vi "Actor Core.vi"(8 "error in":errorcluster, 11 "DataBase in":refnum<class "DataBase.lvclass">) -> (0 "error out":errorcluster, 3 "Actor out":refnum<class "Actor.lvclass">)   [LabVIEW 2019, in "DataBase.lvlib" / "DataBase.lvclass"]
doc: "(<B>Filename</B>: Actor Framework.lvlib:Actor.lvclass:Actor Core.vi)\n\nReceives messages to the actor, reacts to them, and initiates any error handling that may shut the actor down.\n\nDescendant classes may override this VI to append parallel tasks for the actor to complete while it handles messages. Overrides use the Call Parent Class Method node."
uses:
  DataBase.lvclass
  C:/Program Files (x86)/National Instruments/LabVIEW 2019/vi.lib/ActorFramework/Actor/Actor.lvclass
  <vilib>/ActorFramework/Actor/Actor.lvclass
  DataBase.lvclass/DataBase.ctl
  <vilib>/ActorFramework/Actor/Actor.lvclass/Actor.ctl
  <vilib>/ActorFramework/Message Enqueuer/Message Enqueuer.lvclass/Message Enqueuer.ctl
  <vilib>/ActorFramework/Message Enqueuer/Init from Existing Queue.vi
  <vilib>/ActorFramework/Message Enqueuer/Enqueue.vi
  DataBase Messages/SelectData Msg/SelectData Msg.lvclass
  C:/Program Files (x86)/National Instruments/LabVIEW 2019/vi.lib/ActorFramework/Message/Message.lvclass
  DataBase Messages/NextPage Msg/NextPage Msg.lvclass
  DataBase Messages/PreviousPage Msg/PreviousPage Msg.lvclass
  DataBase Messages/Export Msg/Export Msg.lvclass
  DataBase Messages/SearchSerialNumber Msg/SearchSerialNumber Msg.lvclass
  DataBase Messages/ShowDetailResult Msg/ShowDetailResult Msg.lvclass
  <vilib>/ActorFramework/Message Priority Queue/Priority Enqueue.vi
  <vilib>/NI/Event Source Actor/Event Source/Event Source/Event Source.lvclass
  <vilib>/ActorFramework/Message Enqueuer/Message Enqueuer.lvclass
panel:
  in  "Station":T1(ring)
  in  "TableName":string(combo)
  in  "Radio Buttons":enum32{"PDF", "Excel"}(radio)=enum."Excel"
  in  "ShowDetail":bool
  in  "Search":bool
  in  "SerialNumber":string
  in  "TimeRange":T2(ring)
  in  "Export":bool
  in  "StartTime":timestamp=timestamp(3714617125.102728 s since 1904-01-01) format="%<%x>T"
  in  "PreviousPage":bool
  in  "NextPage":bool
  in  "Multicolumn Listbox":i32(listbox)
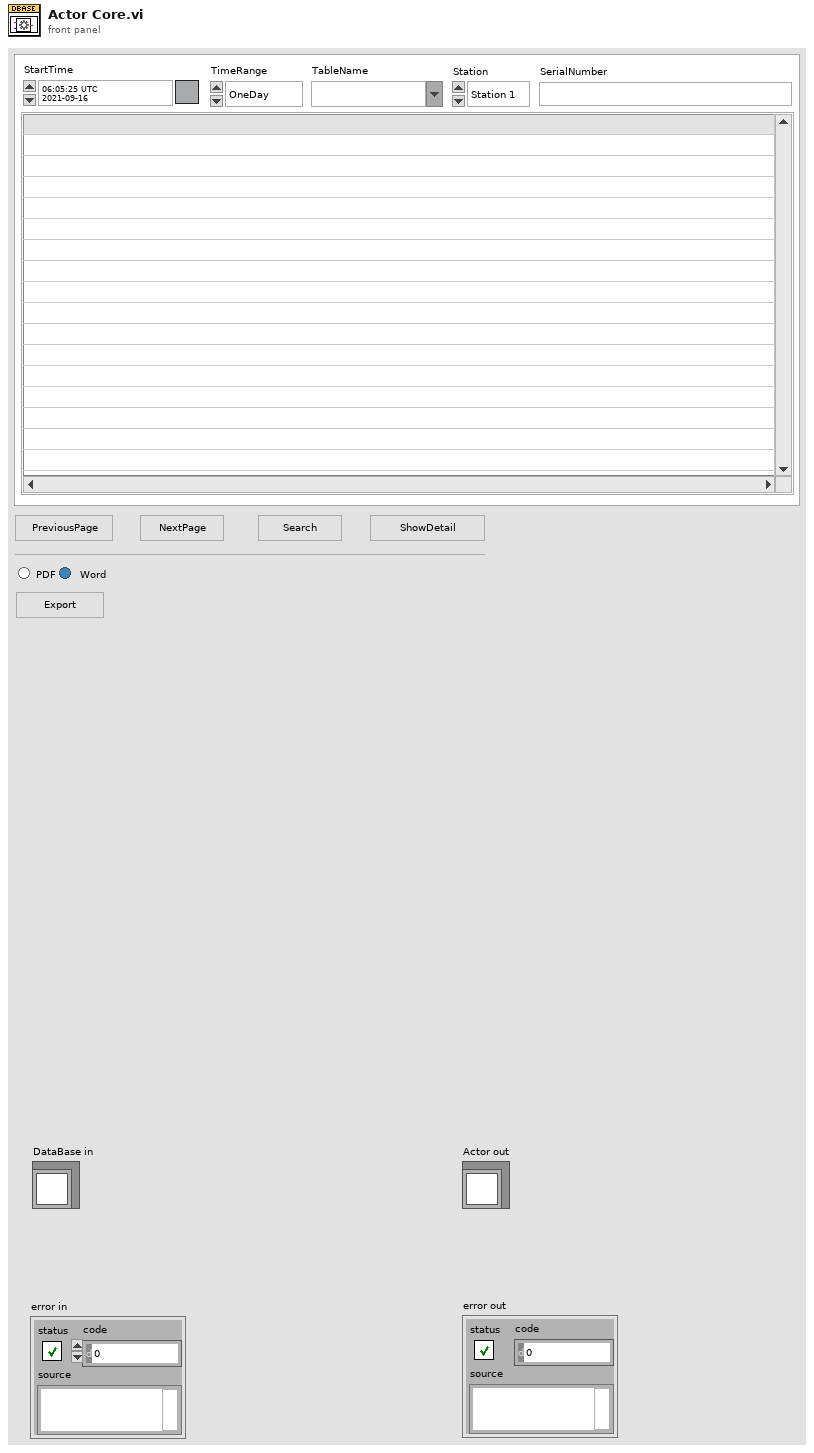
[diagram p1: front panel]
types:
  T1 = enum16{"Station 1", "Station 2", "Station 3", "Station 4"}
  T2 = enum16{"OneDay", "OneWeek", "OneMonth", "OneYear"}
  T3 = enum32{"Invalid", "Standard", "Closed", "Hidden", "Minimized", "Maximized"}
  T4 = enum32{"invalid app kind", "Development System", "Run Time System", "Student Edition", "Embedded LabVIEW", "Evaluation", "Custom"}
  T5 = cluster{"Core":cluster{"Current VI Reference":refnum<vi>, "Close Panel on Exit?":bool}, "Your Boolean data":bool, "Your string data":string}
  T6 = cluster{"Current VI Reference":refnum<vi>, "Close Panel on Exit?":bool}
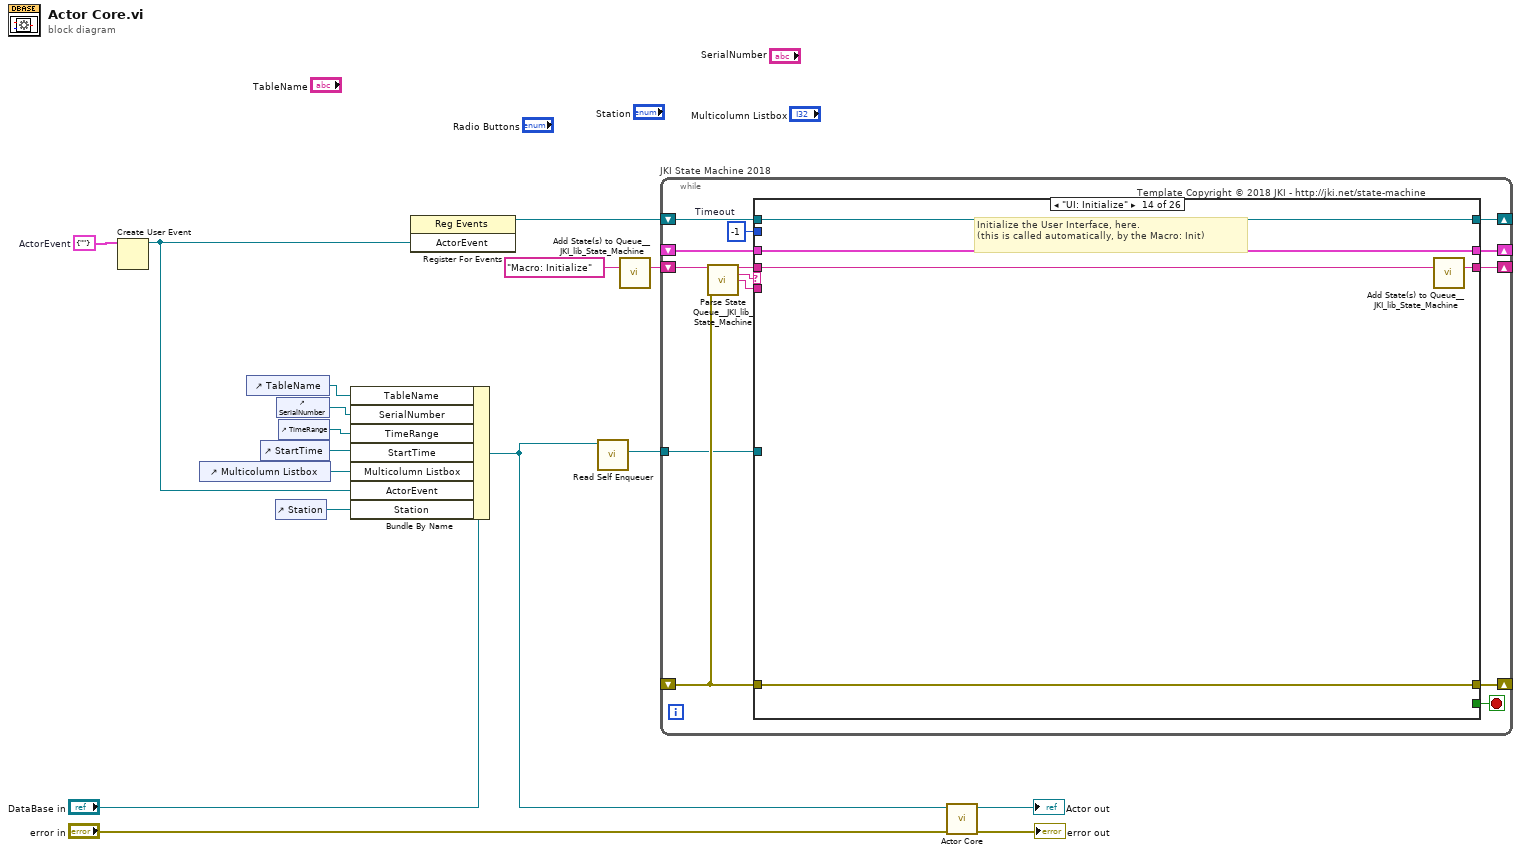
[diagram p0: block diagram]
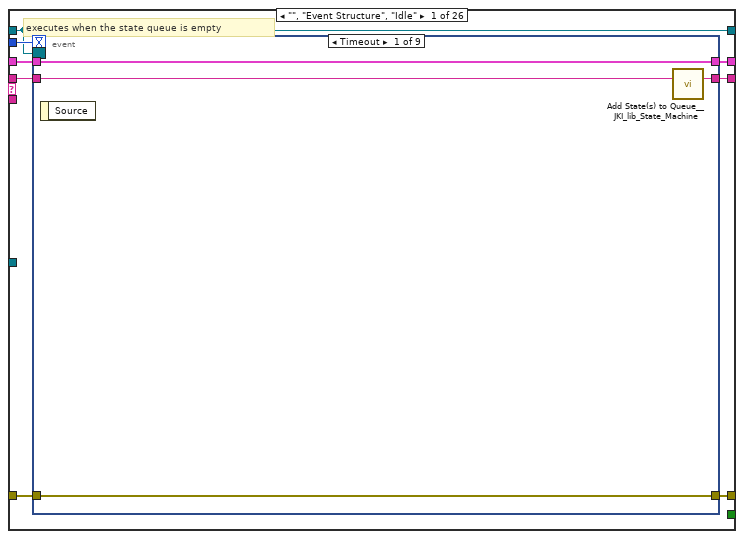
[diagram p2: hidden frame]
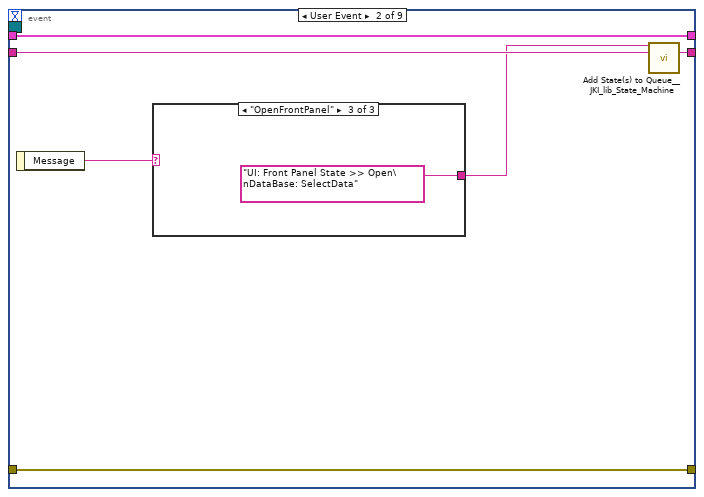
[diagram p3: hidden frame]
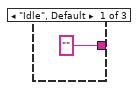
[diagram p4: hidden frame]
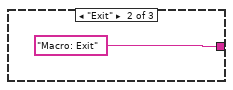
[diagram p5: hidden frame]
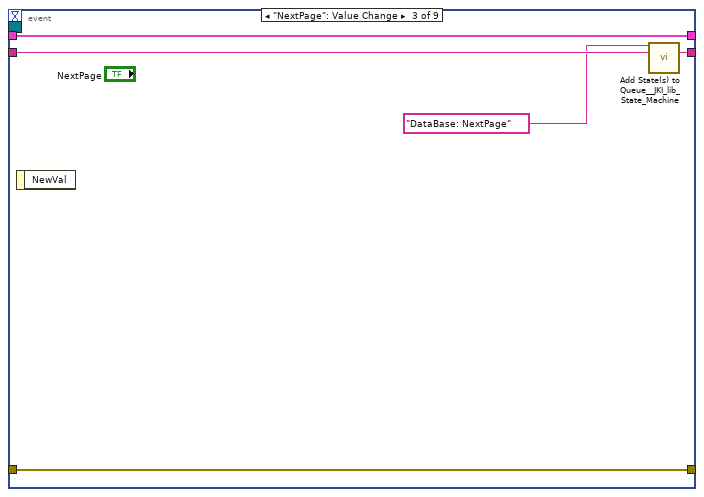
[diagram p6: hidden frame]
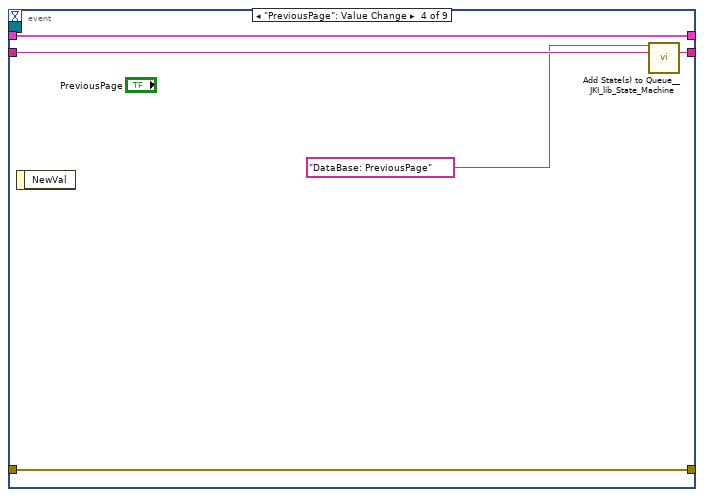
[diagram p7: hidden frame]
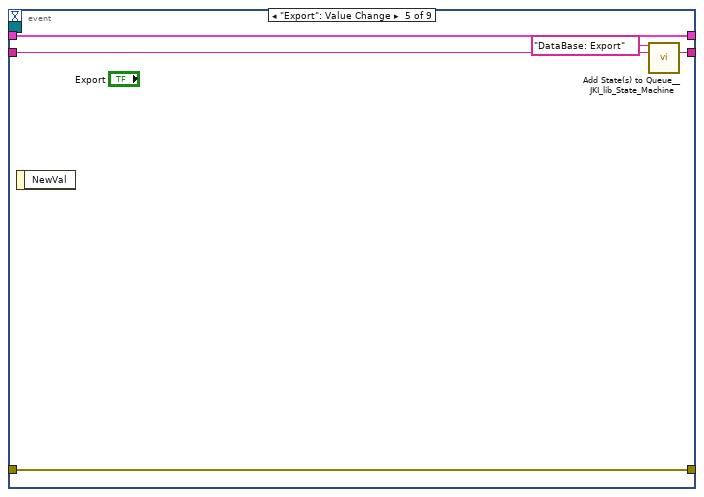
[diagram p8: hidden frame]
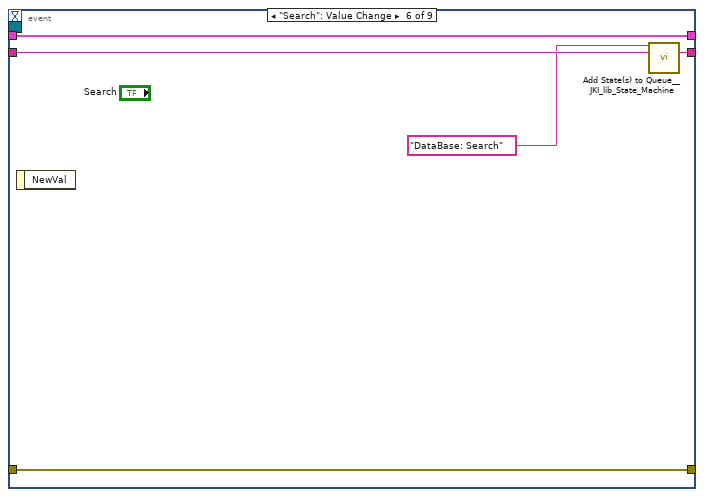
[diagram p9: hidden frame]
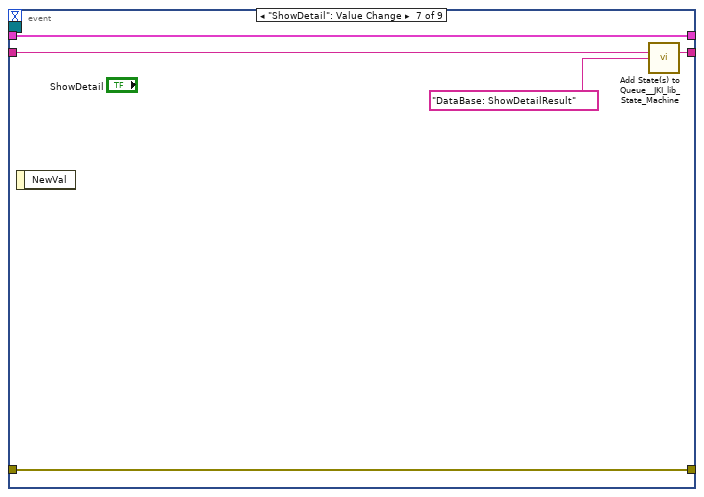
[diagram p10: hidden frame]
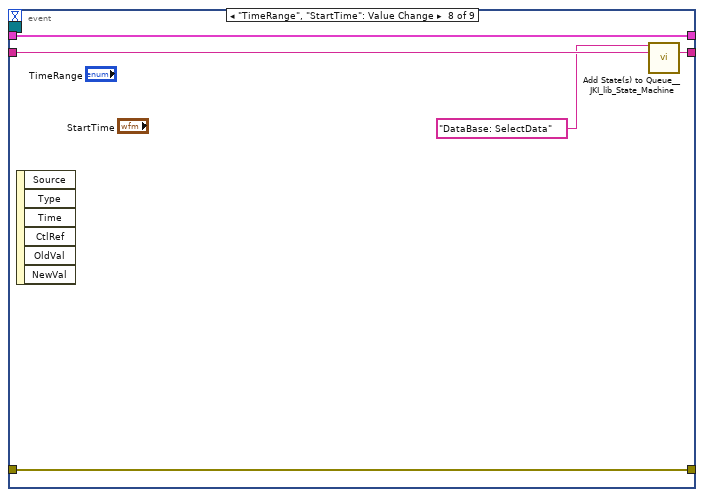
[diagram p11: hidden frame]
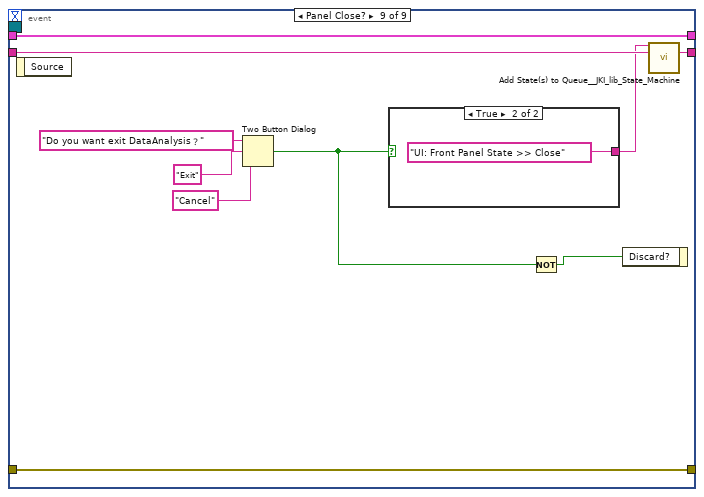
[diagram p12: hidden frame]
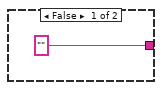
[diagram p13: hidden frame]
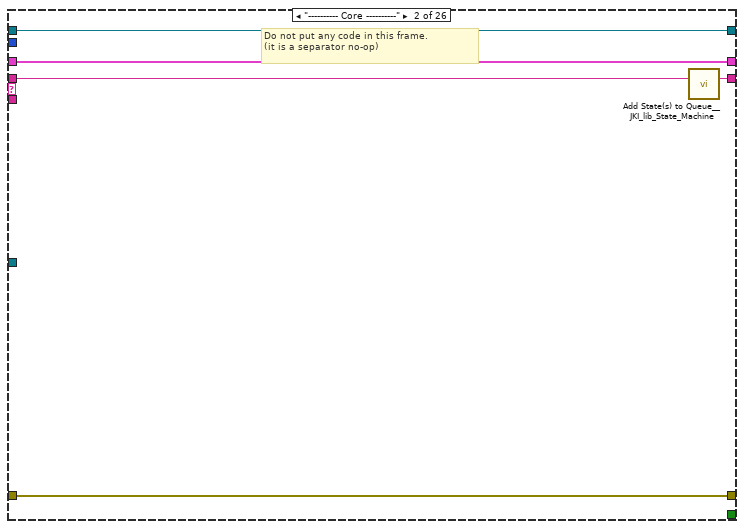
[diagram p14: hidden frame]
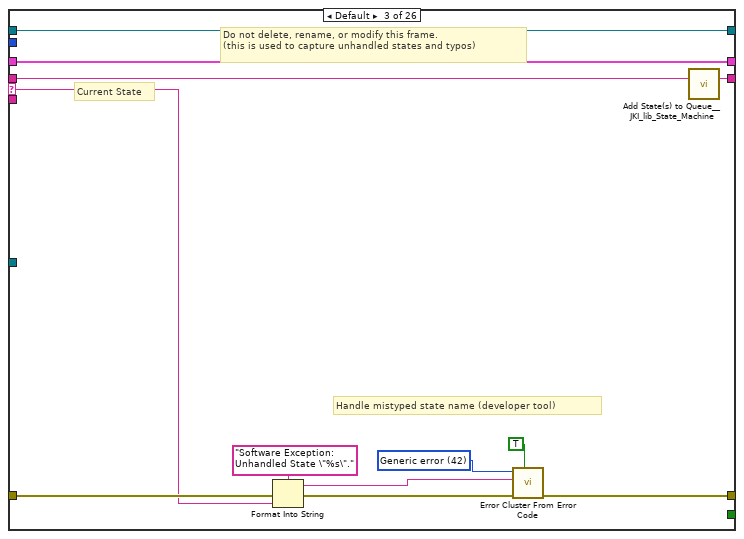
[diagram p15: hidden frame]
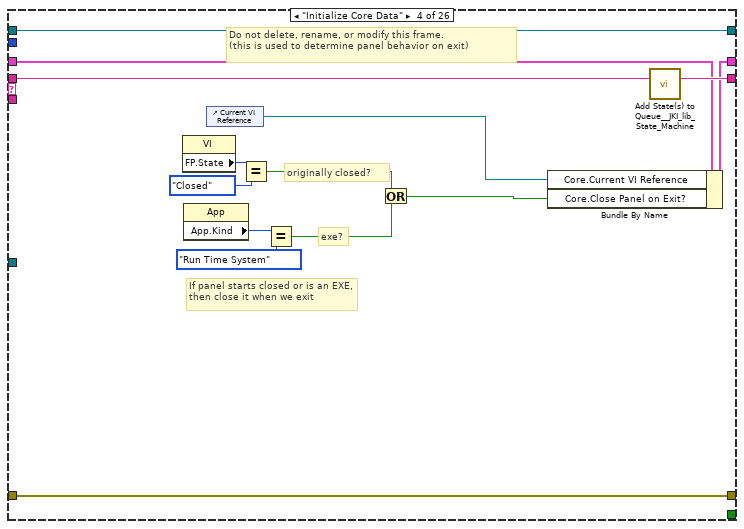
[diagram p16: hidden frame]
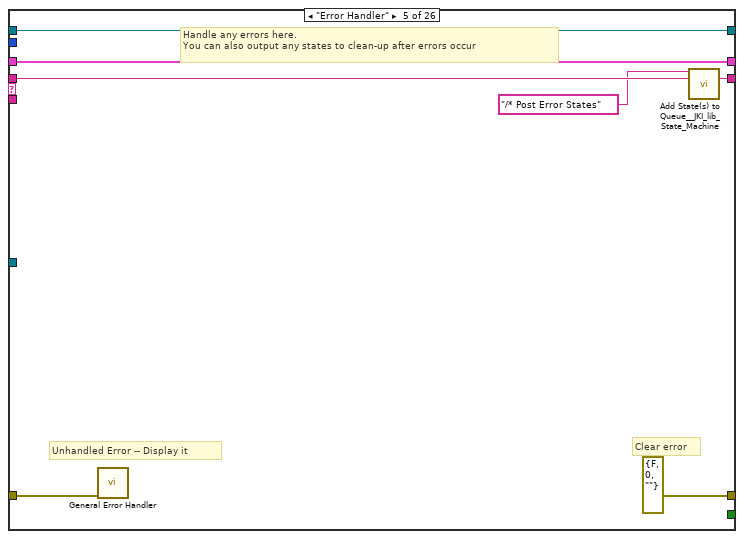
[diagram p17: hidden frame]
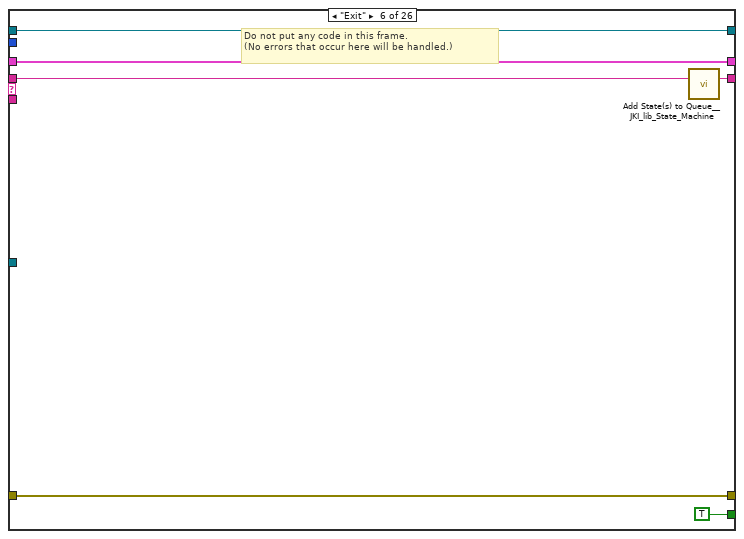
[diagram p18: hidden frame]
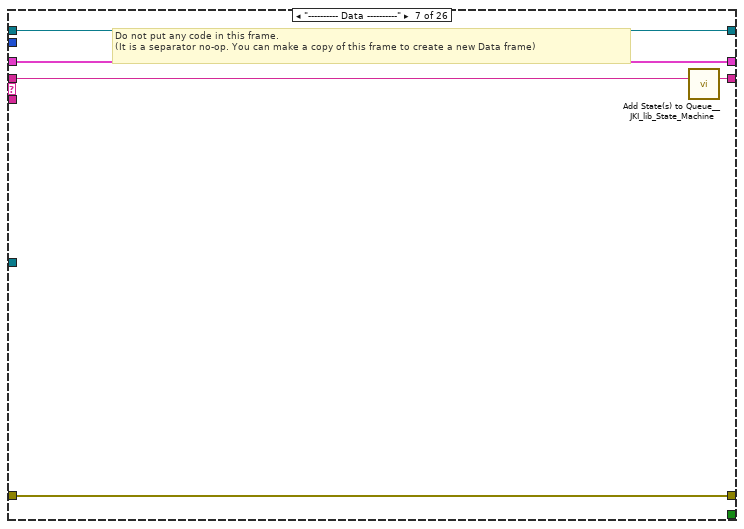
[diagram p19: hidden frame]
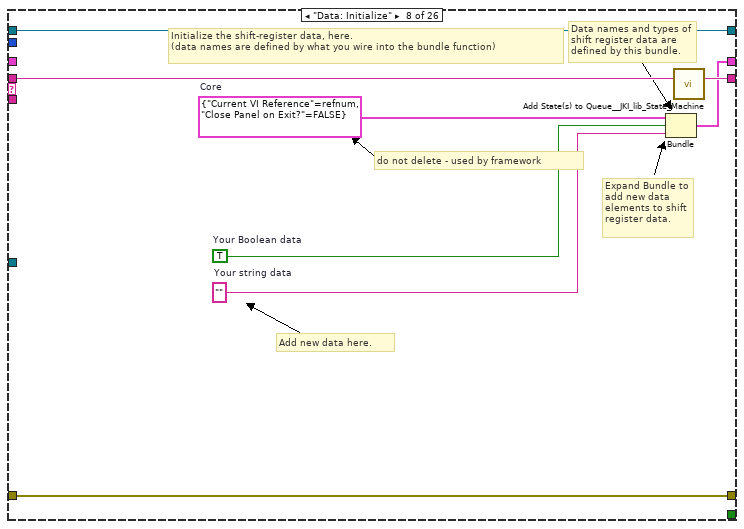
[diagram p20: hidden frame]
diagram:
  w11 = cluster{"Message":string} {"Message"=""}  # ActorEvent
  n1 = Create User Event(user event datatype=w11) -> (user event=w9:refnum<user-event>)  [unwired: 1 in, 1 out]
  n2 = control-ref of="Multicolumn Listbox"() -> (w7:refnum<vi>)
  n3 = control-ref of="TableName"() -> (w2:refnum<vi>)
  n4 = control-ref of="StartTime"() -> (w6:refnum<vi>)
  n5 = control-ref of="Station"() -> (w1:refnum<vi>)
  n6 = control-ref of="SerialNumber"() -> (w3:refnum<vi>)
  n7 = control-ref of="TimeRange"() -> (w5:refnum<vi>)
  n8 = Bundle By Name(cluster="DataBase in", "TableName"=w2, "SerialNumber"=w3, "TimeRange"=w5, "StartTime"=w6, "Multicolumn Listbox"=w7, "ActorEvent"=w9, "Station"=w1) -> (w4:refnum<class "DataBase.lvclass">)
  n9 = register-events(w9) -> (reference out=w12:refnum<event-registration>)  [unwired: 2 in, 1 out]
  n10 = call <vilib>:"Read Self Enqueuer.vi"("Actor"=w4) -> ("Self Enqueuer"=w8:refnum<class "Message Enqueuer.lvclass">)  [unwired: 10 in]
  n11 = call <vilib>:"Add State(s) to Queue__JKI_lib_State_Machine.vi"("State(s) in (\"\")"="Macro: Initialize") -> ("States Out"=w14:string)  [unwired: 14 in]
  n12 = while "JKI State Machine 2018" {
    shift-right: [w24] -> _
    shift-left: _ -> [w23]
    shift-right: [w27] -> _
    shift-left: _ -> [w21]
    shift-right: [w26] -> _
    shift-left: w14 -> [w28]
    shift-right: [w20] -> _
    shift-left: w12 -> [w19]
    tunnel: w8 -> [w18]
    stop <- w25 stop-if-true
    w22 = -1  # Timeout
    # "Template Copyright © 2018 JKI - http://jki.net/state-machine"
    n13 = call <vilib>:"Parse State Queue__JKI_lib_State_Machine.vi"("State Queue"=w28, "Error In (no error)"=w21) -> ("Remaining States"=w30:string, "Current State"=w31:string, "Arguments"=w29:string)  [unwired: 11 in]
    n14 = case shown="\"UI: Initialize\"" w31 {
      selector: w31 -> [_ _ w101 _ _ _ _ _ _ _ _ _ _ _ _ _ _ _ _ _ _ _ _ _ _ _]
      tunnel: w30 -> [w39 w99 w105 w125 w132 w138 w143 w151 w158 w163 w168 w174 w179 w184 w191 w203 w273 w279 w290 w295 w302 w308 w314 w320 w326 w332]
      tunnel: w29 -> [_ _ _ _ _ _ _ _ _ _ _ _ _ _ w186 w197 _ _ _ _ _ _ _ _ _ _]
      tunnel: w23 -> [w37 w96 w103 w118 w129 w136 w140 _ w153 w160 w166 w172 w176 w182 w189 w199 w270 w276 w287 w292 w300 w305 w311 w317 w323 w329]
      tunnel: [w36 w97 w107 w122 errorcluster {"status"=FALSE, "code"=0, "source"=""} ("error out") w135 w141 w148 w154 w161 w165 w169 w177 w181 w187 w200 w271 w277 w288 w293 w297 w306 w312 w318 w324 w330] -> w27
      tunnel: w21 -> [w35 w97 w106 w122 w128 w135 w141 w148 w155 w161 w165 w170 w177 w181 w188 w201 w271 w277 w288 w293 w297 w306 w312 w318 w324 w330]
      tunnel: [w38 w98 w104 w124 w131 w137 w142 w150 w157 w162 w167 w173 w178 w183 w190 w202 w272 w278 w289 w294 w301 w307 w313 w319 w325 w331] -> w26
      tunnel: [_ _ _ _ _ TRUE _ _ _ _ _ _ _ _ _ _ _ _ _ _ _ _ _ _ _ _] -> w25
      tunnel: [w34 w96 w103 w123 w129 w136 w140 w149 w153 w160 w166 w172 w176 w182 w189 w199 w270 w276 w287 w292 w300 w305 w311 w317 w323 w329] -> w24
      tunnel: w22 -> [w33 _ _ _ _ _ _ _ _ _ _ _ _ _ _ _ _ _ _ _ _ _ _ _ _ _]
      tunnel: [w32 w95 w100 w112 w126 w133 w139 w144 w152 w159 w164 w171 w175 w180 w185 w196 w269 w274 w280 w291 w299 w304 w310 w316 w322 w328] -> w20
      tunnel: w19 -> [w32 w95 w100 w112 w126 w133 w139 w144 w152 w159 w164 w171 w175 w180 w185 w196 w269 w274 w280 w291 w299 w304 w310 w316 w322 w328]
      tunnel: w18 -> [_ _ _ _ _ _ _ _ _ _ _ _ _ _ _ _ _ _ _ _ w298 w303 w309 w315 w321 w327]
      frame "", "Event Structure", "Idle" {
        # "executes when the state queue is empty"
        n15 = event shown="[0] Timeout" {
          selector: w32 -> [_ _ _ _ _ _ _ _ _]
          dyn-events: _ -> [_ _ _ _ _ _ _ _ _]
          timeout: w33 -> [_ _ _ _ _ _ _ _ _]
          tunnel: w39 -> [w43 w49 w57 w62 w67 w72 w77 w82 w92]
          tunnel: [w42 w48 w56 w61 w66 w71 w76 w81 w91] -> w38
          tunnel: w37 -> [w40 w46 w54 w59 w64 w69 w74 w79 w89]
          tunnel: [w41 w47 w55 w60 w65 w70 w75 w80 w90] -> w36
          tunnel: w35 -> [w41 w47 w55 w60 w65 w70 w75 w80 w90]
          tunnel: [w40 w46 w54 w59 w64 w69 w74 w79 w89] -> w34
          event Timeout {
            n16 = event-data() -> ()  [unwired: 1 in, 1 out]
            n17 = call <vilib>:"Add State(s) to Queue__JKI_lib_State_Machine.vi"("State(s) in (\"\")"=w43) -> ("States Out"=w42:string)  [unwired: 14 in]
          }
          event User Event {
            n18 = event-data() -> ("Message"=w45:string)  [unwired: 1 in]
            n19 = case shown="\"OpenFrontPanel\"" w45 {
              tunnel: ["" "Macro: Exit" "UI: Front Panel State >> Open\nDataBase: SelectData"] -> w44
              frame "Idle", Default {
              }
              frame "Exit" {
              }
              frame "OpenFrontPanel" {
              }
            }
            n20 = call <vilib>:"Add State(s) to Queue__JKI_lib_State_Machine.vi"("State(s) in Front (\"\")"=w44, "State(s) in (\"\")"=w49) -> ("States Out"=w48:string)  [unwired: 13 in]
          }
          event "NextPage": Value Change {
            n21 = event-data() -> ()  [unwired: 1 in, 1 out]
            n22 = call <vilib>:"Add State(s) to Queue__JKI_lib_State_Machine.vi"("State(s) in Front (\"\")"="DataBase: NextPage" ("State(s) in Front (\"\")"), "State(s) in (\"\")"=w57) -> ("States Out"=w56:string)  [unwired: 13 in]
          }
          event "PreviousPage": Value Change {
            n23 = event-data() -> ()  [unwired: 1 in, 1 out]
            n24 = call <vilib>:"Add State(s) to Queue__JKI_lib_State_Machine.vi"("State(s) in Front (\"\")"="DataBase: PreviousPage" ("State(s) in Front (\"\")"), "State(s) in (\"\")"=w62) -> ("States Out"=w61:string)  [unwired: 13 in]
          }
          event "Export": Value Change {
            n25 = event-data() -> ()  [unwired: 1 in, 1 out]
            n26 = call <vilib>:"Add State(s) to Queue__JKI_lib_State_Machine.vi"("State(s) in Front (\"\")"="DataBase: Export" ("State(s) in Front (\"\")"), "State(s) in (\"\")"=w67) -> ("States Out"=w66:string)  [unwired: 13 in]
          }
          event "Search": Value Change {
            n27 = event-data() -> ()  [unwired: 1 in, 1 out]
            n28 = call <vilib>:"Add State(s) to Queue__JKI_lib_State_Machine.vi"("State(s) in Front (\"\")"="DataBase: Search" ("State(s) in Front (\"\")"), "State(s) in (\"\")"=w72) -> ("States Out"=w71:string)  [unwired: 13 in]
          }
          event "ShowDetail": Value Change {
            n29 = event-data() -> ()  [unwired: 1 in, 1 out]
            n30 = call <vilib>:"Add State(s) to Queue__JKI_lib_State_Machine.vi"("State(s) in (\"\")"=w77, "State(s) at Back (\"\")"="DataBase: ShowDetailResult" ("State(s) at Back (\"\")")) -> ("States Out"=w76:string)  [unwired: 13 in]
          }
          event "TimeRange", "StartTime": Value Change {
            n31 = event-data() -> ()  [unwired: 1 in, 6 out]
            n32 = call <vilib>:"Add State(s) to Queue__JKI_lib_State_Machine.vi"("State(s) in Front (\"\")"="DataBase: SelectData" ("State(s) in Front (\"\")"), "State(s) in (\"\")"=w82) -> ("States Out"=w81:string)  [unwired: 13 in]
          }
          event Panel Close? {
            n33 = event-data() -> ()  [unwired: 1 in, 1 out]
            n34 = Two Button Dialog(message="Do you want exit DataAnalysis？", 1:"Cancel" ("F button name (\"Cancel\")"), 2:"Exit" ("T button name (\"OK\")")) -> (T button?=w86:bool)
            n35 = case shown="True" w86 {
              tunnel: ["" "UI: Front Panel State >> Close"] -> w83
              frame False {
              }
              frame True {
              }
            }
            n36 = Not(x=w86) -> (.not. x?=w84:bool)
            n37 = event-data("Discard?"=w84) -> ()  [unwired: 1 in, 1 out]
            n38 = call <vilib>:"Add State(s) to Queue__JKI_lib_State_Machine.vi"("State(s) in Front (\"\")"=w83, "State(s) in (\"\")"=w92) -> ("States Out"=w91:string)  [unwired: 13 in]
          }
        }
      }
      frame "---------- Core ----------" {
        # "Do not put any code in this frame.\n(it is a separator no-op)"
        n39 = call <vilib>:"Add State(s) to Queue__JKI_lib_State_Machine.vi"("State(s) in (\"\")"=w99) -> ("States Out"=w98:string)  [unwired: 14 in]
      }
      frame Default {
        w110 = 42 items=["No error", "Argument error", "Memory is full", "Out of zone", "End of file", "File already open", "Generic file I/O error", "File not found", "File permission error", "Disk is full", "Duplicate path", "Too many files open", "System feature not enabled", "Resource file not found", "Cannot add resource", "Resource not found", "Image not found", "Image memory error", "Pen does not exist", "Config type invalid", "Config token not found", "Config parse error", "Config memory error", "Bad external code format", "Bad external code offset", "External code not present", "Null window", "Destroy window error", "Null menu", "Print aborted", "Bad print record", "Print driver error", "Windows error during printing", "Memory error during printing", "Print dialog error", "Generic print error", "Invalid device refnum", "Device not found", "Device parameter error", "Device unit error", "Cannot open device", "Device call aborted", "Generic error", "Cancelled by user", "Object ID too low", "Object ID too high", "Object not in heap", "Unknown heap", "Unknown object (invalid DefProc)", "Unknown object (DefProc not in table)", "Message out of range", "Invalid (null) method", "Unknown message", "Manager call not supported", "Bad address", "Network operation in progress", "Network operation timed out", "Connection is busy", "Network attribute not supported", "Network error", "Address in use", "System out of memory", "Connection aborted", "Connection refused", "Not connected", "Already connected", "Connection closed", "Initialization error (interapplication manager)", "Bad occurrence", "Wait on unbound occurrence handler", "Occurrence queue overflow", "Datalog type conflict", "Unused", "Unrecognized type (interapplication manager)", "Memory corrupt", "Failed to make temporary DLL", "Old CIN version", "Drag socket not found", "Failed to load drop-object", "Failed to register OLE object", "Failed to release OLE object", "Format specifier type mismatch", "Unknown format specifier", "Too few format specifiers", "Too many format specifiers", "Scan failed", "Newer CIN version", "Error converting to variant", "Runtime menu error", "Password tampered", "Variant attribute not found", "Incompatible variant data type", "Event data is not available", "Event Store is not present", "Occurrence is not found", "Event Queue is not created", "Event info is not available", "Refnum passed is NULL", "Error retrieving Class GUID", "Error retrieving CoClass GUID", "Error retrieving TypeLib GUID.", "Bad built application magic bytes.", "Specific driver is different from the specific driver associated with the Logical Name.", "There is no session opened to the class driver.", "Max Error", "MAX - Error with config objects", "MAX - Error loading configuration", "MAX - Group not supported"]
        # "Current State"
        # "Do not delete, rename, or modify this frame.\n(this is used to capture unhandled states and typos)"
        # "Handle mistyped state name (developer tool)"
        n40 = Format Into String(format string="Software Exception: Unhandled State \"%s\"." ("message"), error in=w106, w101) -> (resulting string=w109:string, error out=w108:errorcluster)  [unwired: 1 in]
        n41 = call <vilib>:"Error Cluster From Error Code.vi"("show call chain? (False)"=TRUE, "error in (no error)"=w108, "error message (\"\")"=w109, "error code (0)"=w110) -> ("error out"=w107:errorcluster)  [unwired: 5 in]
        n42 = call <vilib>:"Add State(s) to Queue__JKI_lib_State_Machine.vi"("State(s) in (\"\")"=w105) -> ("States Out"=w104:string)  [unwired: 14 in]
      }
      frame "Initialize Core Data" {
        # "Do not delete, rename, or modify this frame.\n(this is used to determine panel behavior on exit)"
        # "originally closed?"
        # "exe?"
        # "If panel starts closed or is an EXE, then close it when we exit"
        n43 = property class="VI"() -> ("FP.State"=w115:T3)  [unwired: 2 in, 2 out]
        n44 = property class="App"() -> ("App.Kind"=w121:T4)  [unwired: 2 in, 2 out]
        n45 = control-ref of="Current VI Reference"() -> (w116:refnum<vi>)
        n46 = Equal?(x=w115, y=T3."Closed" ("Front Panel Window:State")) -> (x = y?=w113:bool)
        n47 = Equal?(x=w121, y=T4."Run Time System" ("Application:Kind")) -> (x = y?=w119:bool)
        n48 = Or(x=w113, y=w119) -> (x .or. y?=w117:bool)
        n49 = Bundle By Name(cluster=w118, "Core.Current VI Reference"=w116, "Core.Close Panel on Exit?"=w117) -> (w123:T5)
        n50 = call <vilib>:"Add State(s) to Queue__JKI_lib_State_Machine.vi"("State(s) in (\"\")"=w125) -> ("States Out"=w124:string)  [unwired: 14 in]
      }
      frame "Error Handler" {
        # "Unhandled Error -- Display it"
        # "Handle any errors here.\nYou can also output any states to clean-up after errors occur"
        # "Clear error"
        n51 = call <vilib>:"General Error Handler.vi"("error in (no error)"=w128) -> ()  [unwired: 10 in, 5 out]
        n52 = call <vilib>:"Add State(s) to Queue__JKI_lib_State_Machine.vi"("State(s) in Front (\"\")"="/* Post Error States", "State(s) in (\"\")"=w132) -> ("States Out"=w131:string)  [unwired: 13 in]
      }
      frame "Exit" {
        # "Do not put any code in this frame.\n(No errors that occur here will be handled.)"
        n53 = call <vilib>:"Add State(s) to Queue__JKI_lib_State_Machine.vi"("State(s) in (\"\")"=w138) -> ("States Out"=w137:string)  [unwired: 14 in]
      }
      frame "---------- Data ----------" {
        # "Do not put any code in this frame.\n(It is a separator no-op. You can make a copy of this frame to create a new Data frame)"
        n54 = call <vilib>:"Add State(s) to Queue__JKI_lib_State_Machine.vi"("State(s) in (\"\")"=w143) -> ("States Out"=w142:string)  [unwired: 14 in]
      }
      frame "Data: Initialize" {
        w145 = T6 {"Current VI Reference"=refnum, "Close Panel on Exit?"=FALSE}  # Core
        w147 = TRUE  # Your Boolean data
        w146 = ""  # Your string data
        # "do not delete - used by framework"
        # "Expand Bundle to add new data elements to shift register data."
        # "Add new data here."
        # "Data names and types of shift register data are defined by this bundle."
        # "Initialize the shift-register data, here.\n(data names are defined by what you wire into the bundle function)"
        n55 = Bundle("Core"=w145, "Your Boolean data"=w147, "Your string data"=w146) -> (w149:T5)  [unwired: 1 in]
        n56 = call <vilib>:"Add State(s) to Queue__JKI_lib_State_Machine.vi"("State(s) in (\"\")"=w151) -> ("States Out"=w150:string)  [unwired: 14 in]
      }
      frame "Data: Cleanup" {
        # "Cleanup any data and references, here.\n(this is called automatically, by the Macro: Exit)"
        n57 = Unbundle By Name(w153) -> ("Core.Current VI Reference"=w156:refnum<vi>)
        n58 = Close Reference(reference=w156, error in (no error)=w155) -> (error out=w154:errorcluster)
        n59 = call <vilib>:"Add State(s) to Queue__JKI_lib_State_Machine.vi"("State(s) in (\"\")"=w158) -> ("States Out"=w157:string)  [unwired: 14 in]
      }
      frame "---------- Events ----------" {
        # "Do not put any code in this frame.\n(It is a separator no-op. You can make a copy of this frame to create a new UI frame)"
        n60 = call <vilib>:"Add State(s) to Queue__JKI_lib_State_Machine.vi"("State(s) in (\"\")"=w163) -> ("States Out"=w162:string)  [unwired: 14 in]
      }
      frame "Events: Register" {
        n61 = call <vilib>:"Add State(s) to Queue__JKI_lib_State_Machine.vi"("State(s) in (\"\")"=w168) -> ("States Out"=w167:string)  [unwired: 14 in]
      }
      frame "Events: Unregister" {
        # "Do not put any code in this frame.\n(It is a separator no-op. You can make a copy of this frame to create a new UI frame)"
        n62 = Unregister For Events(event registration refnum=w171, error in=w170) -> (error out=w169:errorcluster)
        n63 = call <vilib>:"Add State(s) to Queue__JKI_lib_State_Machine.vi"("State(s) in (\"\")"=w174) -> ("States Out"=w173:string)  [unwired: 14 in]
      }
      frame "---------- UI ----------" {
        # "Do not put any code in this frame.\n(It is a separator no-op. You can make a copy of this frame to create a new UI frame)"
        n64 = call <vilib>:"Add State(s) to Queue__JKI_lib_State_Machine.vi"("State(s) in (\"\")"=w179) -> ("States Out"=w178:string)  [unwired: 14 in]
      }
      frame "UI: Initialize" {
        # "Initialize the User Interface, here.\n(this is called automatically, by the Macro: Init)"
        n65 = call <vilib>:"Add State(s) to Queue__JKI_lib_State_Machine.vi"("State(s) in (\"\")"=w184) -> ("States Out"=w183:string)  [unwired: 14 in]
      }
      frame "UI: Cursor Set" {
        # "Argument"
        # "Set and Unset Cursor Busy.\n(Usage: \"UI: Cursor Set >> Busy|Idle\")"
        n66 = case shown="\"Idle\", Default" w186 {
          tunnel: w188 -> [w193 w195]
          tunnel: [w192 w194] -> w187
          frame "Idle", Default {
            n67 = call <vilib>:"Unset Busy.vi"("error in (no error)"=w193) -> ("error out"=w192:errorcluster)  [unwired: 10 in]
          }
          frame "Busy" {
            n68 = call <vilib>:"Set Busy.vi"("error in (no error)"=w195) -> ("error out"=w194:errorcluster)  [unwired: 9 in, 1 out]
          }
        }
        n69 = call <vilib>:"Add State(s) to Queue__JKI_lib_State_Machine.vi"("State(s) in (\"\")"=w191) -> ("States Out"=w190:string)  [unwired: 14 in]
      }
      frame "UI: Front Panel State" {
        # "Argument"
        # "Set Front Panel Open or Closed\n(Usage: \"UI: Front Panel State >> Open|Close\")"
        n70 = Unbundle By Name(w199) -> ("Core.Current VI Reference"=w198:refnum<vi>)
        n71 = case shown="\"Open\", \"Standard\", Default" w197 {
          tunnel: w201 -> [w209 w224 w235 w248 w261]
          tunnel: [w211 w225 w237 w250 w263] -> w200
          tunnel: w198 -> [w210 w222 w236 w249 w262]
          frame "Open", "Standard", Default {
            w204 = T3."Standard" ("State")
            n72 = property class="VI"(reference=w210, error in=w209) -> (reference out=w207:refnum<vi>, error out=w208:errorcluster, "FP.State"=w206:T3)
            n73 = Not Equal?(x=w206, y=w204) -> (x != y?=w205:bool)
            n74 = case shown="True" w205 {
              tunnel: [w215 w217] -> w211
              tunnel: w208 -> [w214 w217]
              tunnel: w207 -> [w213 _]
              tunnel: w204 -> [w212 _]
              frame True {
                n75 = invoke class="VI" method="FP.Open"(reference=w213, error in=w214, "Activate"=TRUE, "State"=w212) -> (error out=w215:errorcluster)  [unwired: 1 in, 4 out]
              }
              frame False {
              }
            }
          }
          frame "Close", "Closed" {
            n76 = property class="VI"(reference=w222, error in=w224) -> (reference out=w221:refnum<vi>, error out=w223:errorcluster, "FP.State"=w219:T3)
            n77 = Not Equal?(x=w219, y=T3."Closed" ("Front Panel Window:State")) -> (x != y?=w218:bool)
            n78 = case shown="True" w218 {
              tunnel: [w226 w229] -> w225
              tunnel: w223 -> [w226 w228]
              tunnel: w221 -> [_ w227]
              frame False {
              }
              frame True {
                n79 = invoke class="VI" method="FP.Close"(reference=w227, error in=w228) -> (error out=w229:errorcluster)  [unwired: 1 in, 2 out]
              }
            }
          }
          frame "Hidden", "Hide" {
            w230 = T3."Hidden" ("State")
            n80 = property class="VI"(reference=w236, error in=w235) -> (reference out=w233:refnum<vi>, error out=w234:errorcluster, "FP.State"=w232:T3)
            n81 = Not Equal?(x=w232, y=w230) -> (x != y?=w231:bool)
            n82 = case shown="True" w231 {
              tunnel: [w241 w242] -> w237
              tunnel: w234 -> [w240 w242]
              tunnel: w233 -> [w239 _]
              tunnel: w230 -> [w238 _]
              frame True {
                n83 = invoke class="VI" method="FP.Open"(reference=w239, error in=w240, "State"=w238) -> (error out=w241:errorcluster)  [unwired: 2 in, 4 out]
              }
              frame False {
              }
            }
          }
          frame "Minimize", "Minimized" {
            w243 = T3."Minimized" ("State")
            n84 = property class="VI"(reference=w249, error in=w248) -> (reference out=w246:refnum<vi>, error out=w247:errorcluster, "FP.State"=w245:T3)
            n85 = Not Equal?(x=w245, y=w243) -> (x != y?=w244:bool)
            n86 = case shown="True" w244 {
              tunnel: [w254 w255] -> w250
              tunnel: w247 -> [w253 w255]
              tunnel: w246 -> [w252 _]
              tunnel: w243 -> [w251 _]
              frame True {
                n87 = invoke class="VI" method="FP.Open"(reference=w252, error in=w253, "State"=w251) -> (error out=w254:errorcluster)  [unwired: 2 in, 4 out]
              }
              frame False {
              }
            }
          }
          frame "Maximize", "Maximized" {
            w256 = T3."Maximized" ("State")
            n88 = property class="VI"(reference=w262, error in=w261) -> (reference out=w259:refnum<vi>, error out=w260:errorcluster, "FP.State"=w258:T3)
            n89 = Not Equal?(x=w258, y=w256) -> (x != y?=w257:bool)
            n90 = case shown="True" w257 {
              tunnel: [w267 w268] -> w263
              tunnel: w260 -> [w266 w268]
              tunnel: w259 -> [w265 _]
              tunnel: w256 -> [w264 _]
              frame True {
                n91 = invoke class="VI" method="FP.Open"(reference=w265, error in=w266, "State"=w264) -> (error out=w267:errorcluster)  [unwired: 2 in, 4 out]
              }
              frame False {
              }
            }
          }
        }
        n92 = call <vilib>:"Add State(s) to Queue__JKI_lib_State_Machine.vi"("State(s) in (\"\")"=w203) -> ("States Out"=w202:string)  [unwired: 14 in]
      }
      frame "---------- Macro ----------" {
        # "Do not put any code in this frame.\n(It is a separator no-op. You can make a copy of this frame to create a new Macro frame)"
        n93 = call <vilib>:"Add State(s) to Queue__JKI_lib_State_Machine.vi"("State(s) in (\"\")"=w273) -> ("States Out"=w272:string)  [unwired: 14 in]
      }
      frame "Macro: Initialize" {
        # "Initialization Macro\n(This is called once, when the VI starts)"
        n94 = call <vilib>:"Add State(s) to Queue__JKI_lib_State_Machine.vi"("State(s) in Front (\"\")"="Data: Initialize\nInitialize Core Data\nEvents: Register\nUI: Initialize\nUI: Front Panel State >> Closed", "State(s) in (\"\")"=w279) -> ("States Out"=w278:string)  [unwired: 13 in]
      }
      frame "Macro: Exit" {
        # "Exit Macro\n(This is called once, when the VI exits)"
        n95 = Unbundle By Name(w287) -> ("Core.Close Panel on Exit?"=w286:bool)
        n96 = Select(t="UI: Front Panel State >> Close", s=w286, f="") -> (s? t:f=w283:string)
        n97 = call <vilib>:"Add State(s) to Queue__JKI_lib_State_Machine.vi"("State(s) in (\"\")"=w283, "State(s) at Back (\"\")"="Data: Cleanup\nEvents: Unregister\nExit") -> ("States Out"=w281:string)  [unwired: 13 in]
        n98 = call <vilib>:"Add State(s) to Queue__JKI_lib_State_Machine.vi"("State(s) in Front (\"\")"=w281, "State(s) in (\"\")"=w290) -> ("States Out"=w289:string)  [unwired: 13 in]
      }
      frame "---------- DataBase ----------" {
        # "Template Separator\n(You can make a copy of, or modify, this frame)"
        n99 = call <vilib>:"Add State(s) to Queue__JKI_lib_State_Machine.vi"("State(s) in (\"\")"=w295) -> ("States Out"=w294:string)  [unwired: 14 in]
      }
      frame "DataBase: SelectData" {
        # "Your code here.\n(You can make a copy of, or modify, this frame)"
        n100 = property on="Multicolumn Listbox" class="MCListbox (strict)"(error in=w297, "Value"=-1 ("Multicolumn Listbox")) -> ()  [unwired: 1 in, 2 out]
        n101 = call "Send SelectData.vi"("Message Enqueuer"=w298) -> ()  [unwired: 9 in, 2 out]
        n102 = call <vilib>:"Add State(s) to Queue__JKI_lib_State_Machine.vi"("State(s) in (\"\")"=w302) -> ("States Out"=w301:string)  [unwired: 14 in]
      }
      frame "DataBase: NextPage" {
        n103 = call "Send NextPage.vi"("Message Enqueuer"=w303) -> ()  [unwired: 9 in, 2 out]
        n104 = call <vilib>:"Add State(s) to Queue__JKI_lib_State_Machine.vi"("State(s) in (\"\")"=w308) -> ("States Out"=w307:string)  [unwired: 14 in]
      }
      frame "DataBase: PreviousPage" {
        n105 = call "Send PreviousPage.vi"("Message Enqueuer"=w309) -> ()  [unwired: 9 in, 2 out]
        n106 = call <vilib>:"Add State(s) to Queue__JKI_lib_State_Machine.vi"("State(s) in (\"\")"=w314) -> ("States Out"=w313:string)  [unwired: 14 in]
      }
      frame "DataBase: Export" {
        n107 = call "Send Export.vi"("Message Enqueuer"=w315) -> ()  [unwired: 9 in, 2 out]
        n108 = call <vilib>:"Add State(s) to Queue__JKI_lib_State_Machine.vi"("State(s) in (\"\")"=w320) -> ("States Out"=w319:string)  [unwired: 14 in]
      }
      frame "DataBase: Search" {
        n109 = call "Send SearchSerialNumber.vi"("Message Enqueuer"=w321) -> ()  [unwired: 9 in, 2 out]
        n110 = call <vilib>:"Add State(s) to Queue__JKI_lib_State_Machine.vi"("State(s) in (\"\")"=w326) -> ("States Out"=w325:string)  [unwired: 14 in]
      }
      frame "DataBase: ShowDetailResult" {
        # "Template Separator\n(You can make a copy of, or modify, this frame)"
        n111 = call "Send ShowDetailResult.vi"("Message Enqueuer"=w327) -> ()  [unwired: 9 in, 2 out]
        n112 = call <vilib>:"Add State(s) to Queue__JKI_lib_State_Machine.vi"("State(s) in (\"\")"=w332) -> ("States Out"=w331:string)  [unwired: 14 in]
      }
    }
  }
  n113 = call-parent "Actor Core.vi"("error in"="error in", "Actor in"=w4) -> ("error out"=→"error out":errorcluster, "Actor out"=→"Actor out":refnum<class "Actor.lvclass">)  [unwired: 8 in]
